vi "Init.vi"(8 "error in (no error)":errorcluster, 9 "Configuration File Path":path=path "", 10 "Name":string, 11 "Execution UI In":refnum<class "Execution UI.lvclass">) -> (0 "error out":errorcluster, 3 "Execution UI Out":refnum<class "Execution UI.lvclass">)   [LabVIEW 2020, in "Execution UI.lvclass"]
uses:
  Execution UI.lvclass
  C:/Git/astemes-lunit/source/Application Framework/Process Classes/Process/Process.lvclass
  Test Runner/Test Runner.lvclass
  Result Collector/Result Collector.lvclass
  Report Generator/Report Generator.lvclass
  Icon Decorator/Icon Decorator.lvclass
  Application Framework/Process Classes/Error Handler/Error Handler.lvclass
  Helper Classes/Buffered Test Finder/Indexing Test Finder.lvclass
  C:/Git/astemes-lunit/source/Framework/Helper Classes/Test Finder/Test Finder.lvclass
  Application Framework/Process Classes/Process/Process.lvclass/Process.ctl
  Report Generator/Report Generator.lvclass/Report Generator.ctl
  Result Collector/Result Collector.lvclass/Result Collector.ctl
  Helper Classes/Buffered Test Finder/Indexing Test Finder.lvclass/Indexing Test Finder.ctl
  Execution UI.lvclass/Execution UI.ctl
  Application Framework/Process Classes/Process/Protected/Messaging/Enqueue Message.vi
  Result Collector/Public/API/Register for Result Events.vi
  Helper Classes/Test Finder/Public/SubVIs/Register For Test Cases Found Event.vi
  Application Framework/Process Classes/Process/Process.lvclass
  C:/Git/astemes-lunit/source/Framework/Helper Classes/Buffered Test Finder/Indexing Test Finder.lvclass
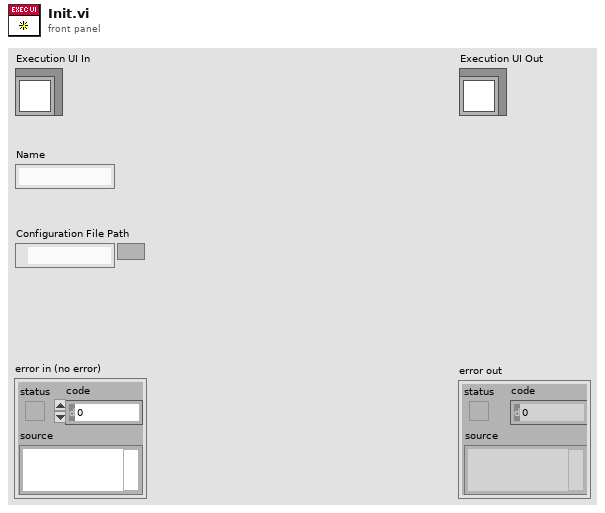
[diagram p1: front panel]
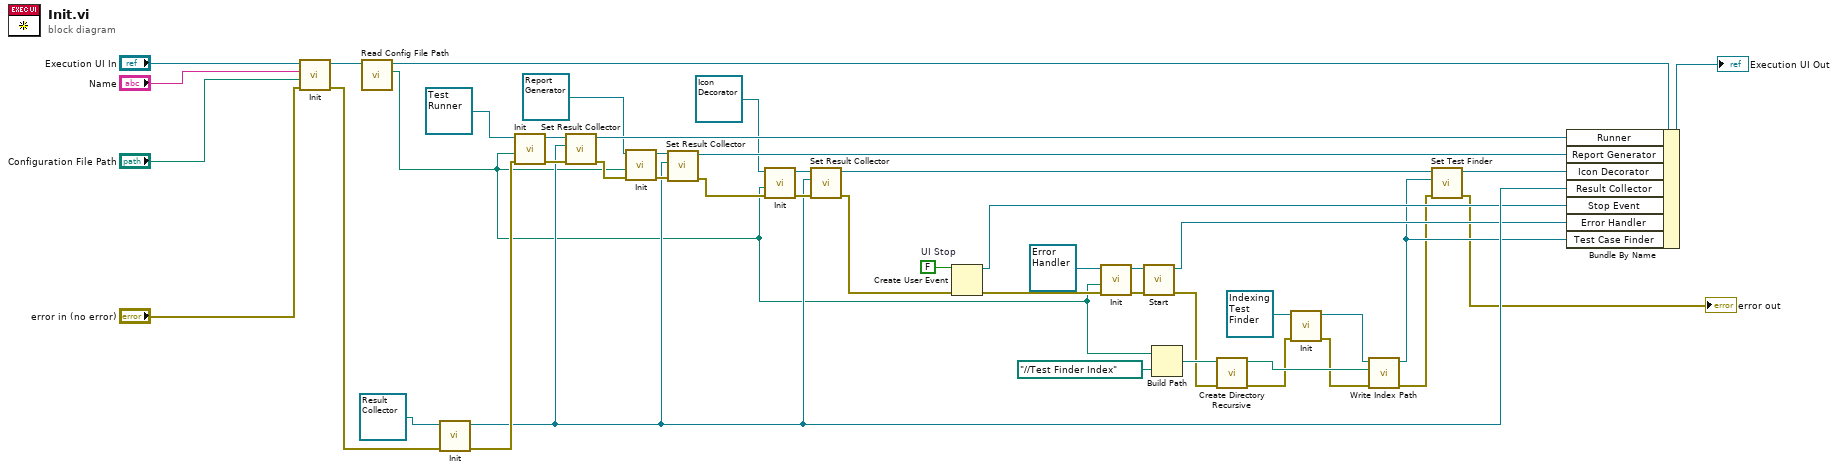
[diagram p0: block diagram]
diagram:
  w24 = FALSE  # UI Stop
  n1 = call-parent "Init.vi"("error in (no error)"="error in (no error)", "Config File Path"="Configuration File Path", "Name"="Name", "Process In"="Execution UI In") -> ("error out"=w42:errorcluster, "Process Out"=w10:refnum<class "Execution UI.lvclass">)  [unwired: 6 in]
  n2 = call "Read Config File Path.vi"("Process In"=w10) -> ("Config File Path"=w8:path, "Process Out"=w9:refnum<class "Execution UI.lvclass">)  [unwired: 8 in, 1 out]
  n3 = call-dynamic "Init.vi"("error in (no error)"=w42, "Report Generator In"=refnum<class "Result Collector.lvclass"> refnum ("Test Report Generator.lvclass")) -> ("error out"=w43:errorcluster, "Report Generator Out"=w25:refnum<class "Result Collector.lvclass">)  [unwired: 8 in]
  n4 = call-dynamic "Init.vi"("error in (no error)"=w43, "Config File Path"=w8, "Test Runner In"=refnum<class "Test Runner.lvclass"> refnum ("Test Runner Spawner.lvclass")) -> ("error out"=w35:errorcluster, "Test Runner Out"=w37:refnum<class "Test Runner.lvclass">)  [unwired: 7 in]
  n5 = call "Set Result Collector.vi"("error in (no error)"=w35, "Result Collector"=w25, "Test Runner In"=w37) -> ("error out"=w30:errorcluster, "Test Runner Out"=w36:refnum<class "Test Runner.lvclass">)  [unwired: 7 in]
  n6 = call-dynamic "Init.vi"("error in (no error)"=w30, "Config File Path"=w8, "Report Generator In"=refnum<class "Report Generator.lvclass"> refnum ("Report Generator.lvclass")) -> ("error out"=w33:errorcluster, "Report Generator Out"=w32:refnum<class "Report Generator.lvclass">)  [unwired: 7 in]
  n7 = call "Set Result Collector.vi"("error in (no error)"=w33, "Result Collector.lvclass"=w25, "Report Generator in"=w32) -> ("error out"=w26:errorcluster, "Report Generator out"=w31:refnum<class "Report Generator.lvclass">)  [unwired: 7 in]
  n8 = call-dynamic "Init.vi"("error in (no error)"=w26, "Config File Path"=w8, "Process In"=refnum<class "Icon Decorator.lvclass"> refnum ("Icon Decorator.lvclass")) -> ("error out"=w27:errorcluster, "Process Out"=w28:refnum<class "Icon Decorator.lvclass">)  [unwired: 7 in]
  n9 = call "Set Result Collector.vi"("error in (no error)"=w27, "Report Generator"=w25, "Icon Decorator In"=w28) -> ("error out"=w1:errorcluster, "Icon Decorator Out"=w6:refnum<class "Icon Decorator.lvclass">)  [unwired: 7 in]
  n10 = Create User Event(user event datatype=w24, error in=w1) -> (user event=w21:refnum<user-event>, error out=w22:errorcluster)
  n11 = call-dynamic "Init.vi"("error in (no error)"=w22, "Configuration File Path"=w8, "Error Handler In"=refnum<class "Error Handler.lvclass"> refnum ("Error Handler in")) -> ("error out"=w18:errorcluster, "Error Handler Out"=w20:refnum<class "Error Handler.lvclass">)  [unwired: 7 in]
  n12 = call "Start.vi"("error in (no error)"=w18, "Process In"=w20) -> ("error out"=w7:errorcluster, "Process Out"=w19:refnum<class "Error Handler.lvclass">)  [unwired: 8 in]
  n13 = Build Path(base path=w8, name or relative path=path "../../Test Finder Index") -> (appended path=w16:path)
  n14 = call <vilib>:"Create Directory Recursive.vi"("error in (no error)"=w7, "directory"=w16) -> ("error out"=w12:errorcluster, "directory copy"=w15:path)  [unwired: 3 in, 1 out]
  n15 = call-dynamic "Init.vi"("error in (no error)"=w12, "Test Finder in"=refnum<class "Indexing Test Finder.lvclass"> refnum ("Indexing Test Finder.lvclass")) -> ("error out"=w11:errorcluster, "Test Finder out"=w13:refnum<class "Indexing Test Finder.lvclass">)  [unwired: 8 in]
  n16 = call "Write Index Path.vi"("error in (no error)"=w11, "Index Folder Path"=w15, "Indexing Test Finder in"=w13) -> ("error out"=w3:errorcluster, "Indexing Test Finder out"=w4:refnum<class "Indexing Test Finder.lvclass">)  [unwired: 7 in]
  n17 = call "Set Test Finder.vi"("error in (no error)"=w3, "Report Generator"=w4, "Icon Decorator In"=w6) -> ("error out"=→"error out":errorcluster, "Icon Decorator Out"=w5:refnum<class "Icon Decorator.lvclass">)  [unwired: 7 in]
  n18 = Bundle By Name(cluster=w9, "Runner"=w36, "Report Generator"=w31, "Icon Decorator"=w5, "Result Collector"=w25, "Stop Event"=w21, "Error Handler"=w19, "Test Case Finder"=w4) -> (→"Execution UI Out":refnum<class "Execution UI.lvclass">)
